vi "setActive.vi"(8 "error in (no error)":errorcluster, 10 "Active?":bool, 11 "IComponent in":refnum<class "IComponent.lvclass">) -> (0 "error out":errorcluster, 3 "IComponent out":refnum<class "IComponent.lvclass">)   [LabVIEW 2022 SP3, in "openDAQ.lvlib" / "IBaseObject.lvlib" / "IPropertyObject.lvlib" / "IComponent.lvlib" / "IComponent.lvclass"]
uses:
  <instrlib>/openDAQ/Public/Classes/IComponent/IComponent.lvclass
  <instrlib>/openDAQ/Public/Classes/IComponent/IComponent.lvclass/IComponent.ctl
  <instrlib>/openDAQ/Binaries/Windows/x86/copendaq32.dll
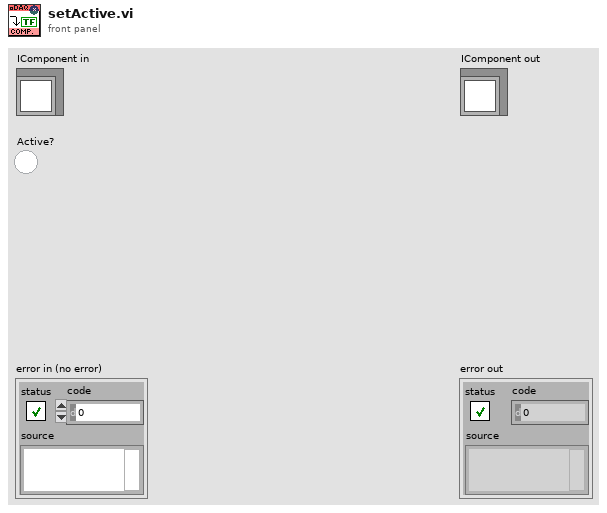
[diagram p1: front panel]
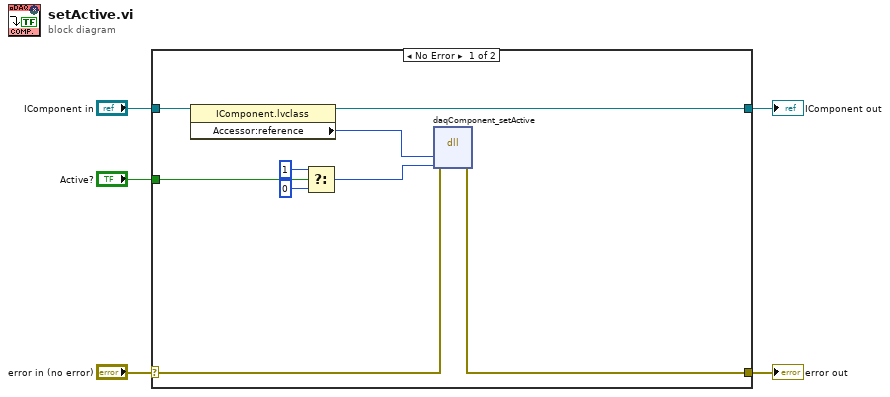
[diagram p0: block diagram]
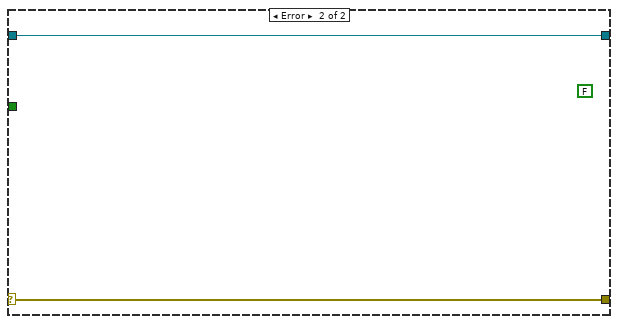
[diagram p2: hidden frame]
diagram:
  n1 = case shown="No Error" "error in (no error)" {
    selector: "error in (no error)" -> [w10 w16]
    tunnel: [w11 w16] -> w4
    tunnel: [w13 w15] -> w2
    tunnel: "IComponent in" -> [w14 w15]
    tunnel: "Active?" -> [w9 _]
    frame No Error {
      n2 = property class="IComponent.lvclass"(reference=w14) -> (reference out=w13:refnum<class "IComponent.lvclass">, "Accessor:reference"=w12:i64)  [unwired: 1 in, 1 out]
      n3 = Select(t=1, s=w9, f=0) -> (s? t:f=w6:i32)
      n4 = dll-call lib="C:/Program Files (x86)/National Instruments/LabVIEW 2022/instr.lib/openDAQ/Binaries/Windows/x86/copendaq*.*" fn="daqComponent_setActive"(error in=w10, "component"=w12, "active"=w6) -> (error out=w11:errorcluster)  [unwired: 5 in, 1 out]
    }
    frame Error {
      (unwired) FALSE
    }
  }
  "error out" <- w4
  "IComponent out" <- w2
